vi "CreateReaderFromClass.vi"(0 "ClassPath/LvClassRef":variant, 5 "error in":errorcluster) -> (10 "Is Interface":bool, 14 "ClassReader":refnum<class "ClassReader.lvclass">, 15 "Description":string, 16 "DataFlowClass":bool, 19 "error out":errorcluster)   [LabVIEW 2020, in "ClassReader.lvclass"]
uses:
  <resource>/Framework/Providers/Open_GDS/ClassProviders/Provider_BaseClassInterface/ClassReader_class/ClassReader.lvclass
  <resource>/Framework/Providers/Open_GDS/ClassProviders/Provider_EndevoGOOP300/ClassReaderGOOP300_class/ClassReaderGOOP300.lvclass
  C:/Program Files (x86)/National Instruments/LabVIEW 2020/resource/Framework/Providers/Open_GDS/ClassProviders/Provider_LvNativeClass/ClassReaderNative_class/ClassReaderNative.lvclass
  <resource>/Framework/Providers/Open_GDS/ClassProviders/Provider_EndevoGOOP400/ClassReaderGOOP400_class/ClassReaderGOOP400.lvclass
  <resource>/Framework/Providers/Open_GDS/ClassProviders/Provider_LvNativeClass/ClassReaderNative_class/ClassReaderNative.lvclass
  C:/Program Files (x86)/National Instruments/LabVIEW 2020/resource/Framework/Providers/Open_GDS/ClassProviders/Provider_BaseClassInterface/ClassReader_class/ClassReader.lvclass
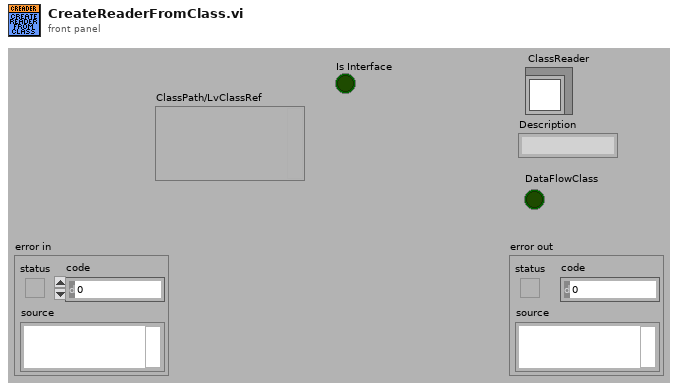
[diagram p1: front panel]
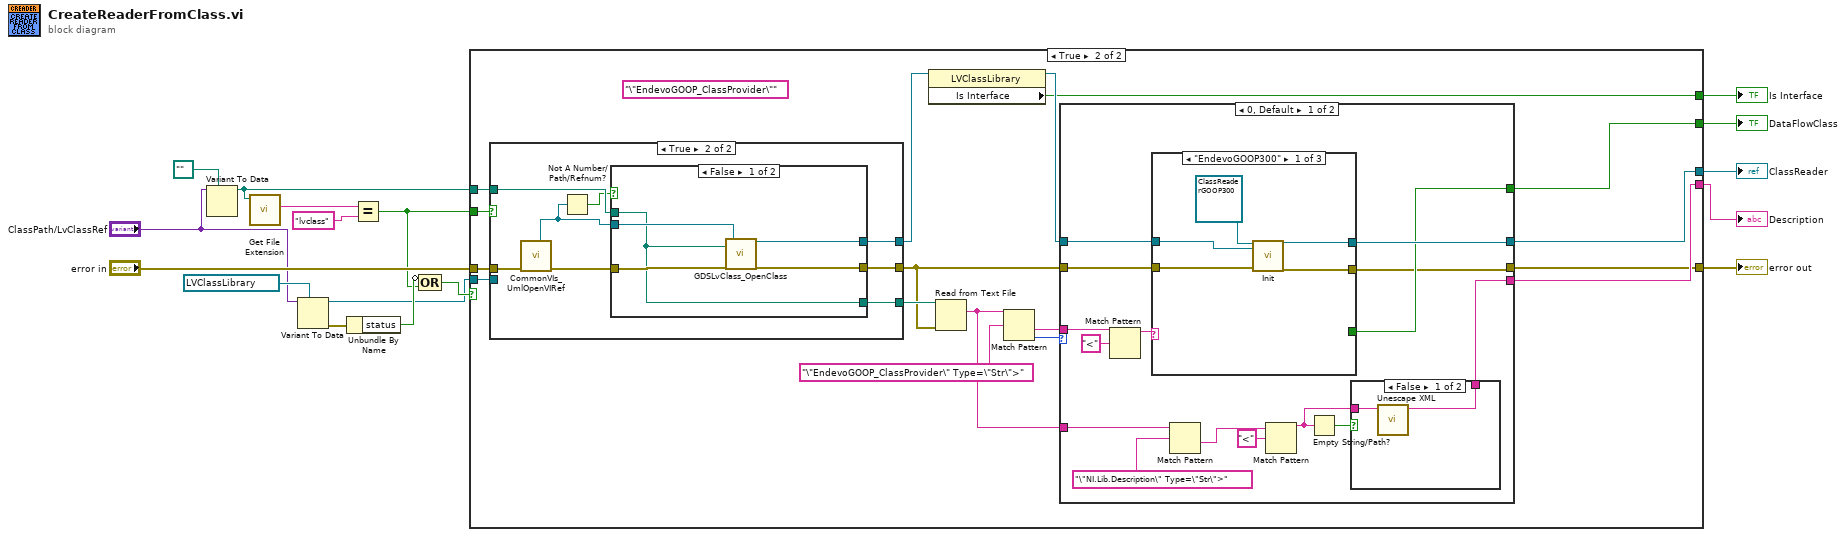
[diagram p0: block diagram]
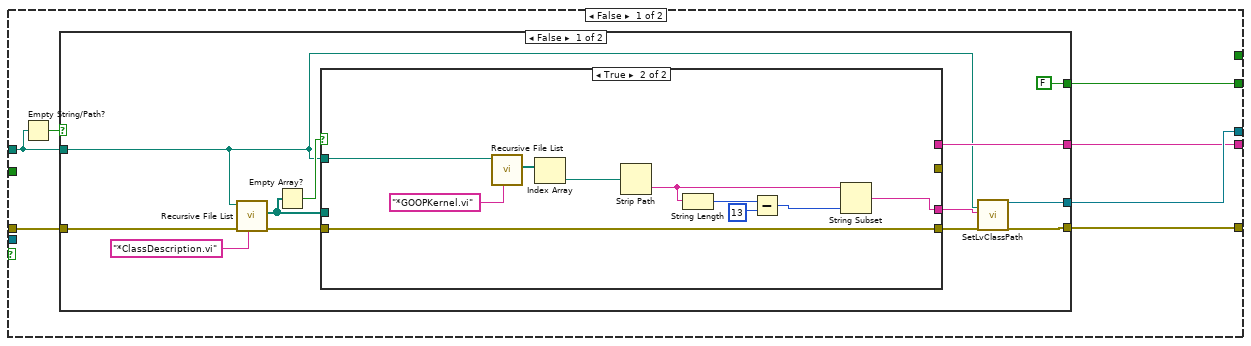
[diagram p2: hidden frame]
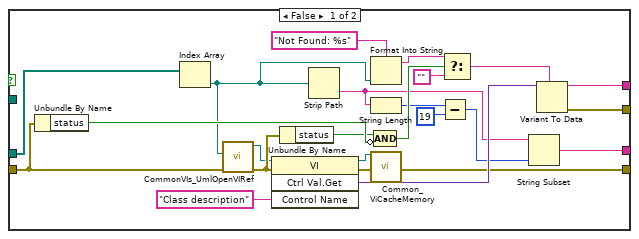
[diagram p3: hidden frame]
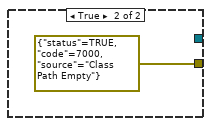
[diagram p4: hidden frame]
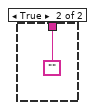
[diagram p5: hidden frame]
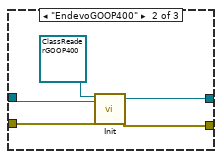
[diagram p6: hidden frame]
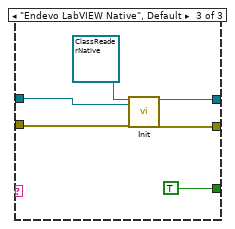
[diagram p7: hidden frame]
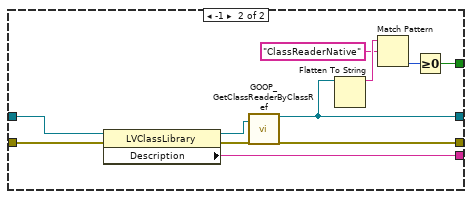
[diagram p8: hidden frame]
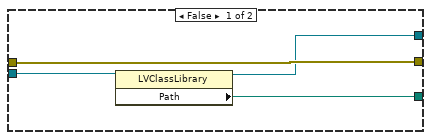
[diagram p9: hidden frame]
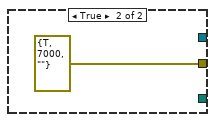
[diagram p10: hidden frame]
diagram:
  n1 = Variant To Data(type=path "", Variant="ClassPath/LvClassRef") -> (data=w5:path)  [unwired: 1 in, 1 out]
  n2 = call <vilib>:"Get File Extension.vi"("file"=w5) -> ("lowercase file extension"=w10:string)  [unwired: 6 in, 4 out]
  n3 = Variant To Data(type=refnum<vi> refnum ("LVClass.Open"), Variant="ClassPath/LvClassRef") -> (data=w4:refnum<vi>, error out=w8:errorcluster)  [unwired: 1 in]
  n4 = Unbundle By Name(w8) -> ("status"=w7:bool)
  n5 = Equal?(x=w10, y="lvclass") -> (x = y?=w3:bool)
  n6 = Compound Arithmetic op=OR(invert w7, w3) -> (w6:bool)
  n7 = case shown="True" w6 {
    tunnel: [w22 w88] -> w17
    tunnel: "error in" -> [w21 w87]
    tunnel: [w24 w82] -> w15
    tunnel: [w23 w86] -> w14
    tunnel: w5 -> [w19 w85]
    tunnel: w4 -> [_ w83]
    tunnel: w3 -> [_ w84]
    tunnel: [w20 w75] -> w2
    tunnel: [_ w72] -> w1
    frame False {
      n8 = Empty String/Path?(string/path=w19) -> (empty?=w18:bool)
      n9 = case shown="False" w18 {
        tunnel: [w36 _] -> w24
        tunnel: [w35 errorcluster {"status"=TRUE, "code"=7000, "source"="Class Path Empty"} ("error out")] -> w23
        tunnel: [w34 _] -> w22
        tunnel: w21 -> [w30 _]
        tunnel: [FALSE _] -> w20
        tunnel: w19 -> [w25 _]
        frame False {
          n10 = call <vilib>:"Recursive File List.vi"("pattern"="*ClassDescription.vi" ("FileSearchPattern"), "error in (no error)"=w30, "Folder Path"=w25) -> ("error out"=w29:errorcluster, "All Files in Dir"=w27:path[])  [unwired: 4 in, 3 out]
          n11 = Empty Array?(array=w27) -> (empty?=w32:bool)
          n12 = case shown="True" w32 {
            tunnel: w29 -> [w46 w70]
            tunnel: [w51 _] -> w34
            tunnel: [w48 w70] -> w33
            tunnel: w27 -> [w47 _]
            tunnel: [w38 w61] -> w31
            tunnel: w25 -> [_ w69]
            tunnel: [w37 _] -> _
            frame False {
              n13 = Unbundle By Name(w46) -> ("status"=w53:bool)
              n14 = Index Array(array=w47) -> (element=w43:path)  [unwired: 1 in]
              n15 = call <resource>:"CommonVIs_UmlOpenVIRef.vi"("error in"=w46, "ViPath/ViName"=w43) -> ("error out"=w45:errorcluster, "vi reference"=w44:refnum<vi>)  [unwired: 6 in, 2 out]
              n16 = invoke class="VI" method="Ctrl Val.Get"(reference=w44, error in=w45, "Control Name"="Class description") -> (reference out=w60:refnum<vi>, error out=w49:errorcluster, "Get Control Value Variant"=w59:variant)  [unwired: 1 in, 1 out]
              n17 = Unbundle By Name(w45) -> ("status"=w52:bool)
              n18 = Strip Path(path=w43) -> (name=w42:string)  [unwired: 1 out]
              n19 = Format Into String(format string="Not Found: %s", w43) -> (resulting string=w57:string)  [unwired: 2 in, 1 out]
              n20 = String Length(string=w42) -> (length=w41:i32)
              n21 = call <resource>:"Common_ ViCacheMemory.vi"("ViRef"=w60, "error in (no error)"=w49) -> ("error out"=w48:errorcluster)  [unwired: 17 in]
              n22 = Compound Arithmetic op=AND(w52, invert w53) -> (w54:bool)
              n23 = Subtract(x=w41, y=19) -> (x-y=w40:i32)
              n24 = Select(t=w57, s=w54, f="") -> (s? t:f=w50:string)
              n25 = String Subset(string=w42, length (rest)=w40) -> (substring=w38:string)  [unwired: 1 in]
              n26 = Variant To Data(type=w50, Variant=w59) -> (data=w51:string, error out=w37:errorcluster)  [unwired: 1 in]
            }
            frame True {
              n27 = call <vilib>:"Recursive File List.vi"("pattern"="*GOOPKernel.vi", "Folder Path"=w69) -> ("All Files in Dir"=w63:path[])  [unwired: 5 in, 4 out]
              n28 = Index Array(array=w63) -> (element=w62:path)  [unwired: 1 in]
              n29 = Strip Path(path=w62) -> (name=w67:string)  [unwired: 1 out]
              n30 = String Length(string=w67) -> (length=w66:i32)
              n31 = Subtract(x=w66, y=13) -> (x-y=w65:i32)
              n32 = String Subset(string=w67, length (rest)=w65) -> (substring=w61:string)  [unwired: 1 in]
            }
          }
          n33 = call <resource>:"SetLvClassPath.vi"("ClassPath"=w25, "ClassName"=w31, "error in (no error)"=w33) -> ("reference out"=w36:refnum<class "ClassReader.lvclass">, "error out"=w35:errorcluster)  [unwired: 15 in]
        }
        frame True {
        }
      }
    }
    frame True {
      (unwired) "\"EndevoGOOP_ClassProvider\"" ("y")
      n34 = case shown="True" w84 {
        tunnel: [w135 w139] -> w74
        tunnel: w87 -> [w137 w145]
        tunnel: [w137 w142] -> w80
        tunnel: w85 -> [_ w143]
        tunnel: w83 -> [w136 _]
        tunnel: [w134 w138] -> w81
        frame False {
          n35 = property class="LVClassLibrary"(reference=w136) -> (reference out=w135:refnum<vi>, "Path"=w134:path)  [unwired: 1 in, 1 out]
        }
        frame True {
          n36 = call <resource>:"CommonVIs_UmlOpenVIRef.vi"("error in"=w145) -> ("error out"=w144:errorcluster, "AppRefOut"=w140:refnum<vi>)  [unwired: 7 in, 2 out]
          n37 = Not A Number/Path/Refnum?(number/path/refnum=w140) -> (NaN/Path/Refnum?=w141:bool)
          n38 = case shown="False" w141 {
            tunnel: [w150 _] -> w139
            tunnel: w144 -> [w149 _]
            tunnel: w143 -> [w146 _]
            tunnel: [w148 errorcluster {"status"=TRUE, "code"=7000, "source"=""} ("error out")] -> w142
            tunnel: w140 -> [w147 _]
            tunnel: [w146 _] -> w138
            frame False {
              n39 = call <resource>:"GDSLvClass_OpenClass.vi"("ClassToOpen"=w146, "error in (no error)"=w149, "Project/ApplicationRef(If empty, currect active project will be used)"=w147) -> ("LVClass.Open"=w150:refnum<vi>, "error out"=w148:errorcluster)  [unwired: 15 in]
            }
            frame True {
            }
          }
        }
      }
      n40 = property class="LVClassLibrary"(reference=w74) -> (reference out=w73:refnum<vi>, "Is Interface"=w72:bool)  [unwired: 1 in, 1 out]
      n41 = Read from Text File(file (use dialog)=w81, error in=w80) -> (text=w76:string)  [unwired: 2 in, 3 out]
      n42 = Match Pattern(string=w76, regular expression="\"EndevoGOOP_ClassProvider\" Type=\"Str\">" ("y")) -> (after substring=w77:string, offset past match=w78:i32)  [unwired: 1 in, 2 out]
      n43 = case shown="0, Default" w78 {
        tunnel: [w94 w133] -> w88
        tunnel: w73 -> [w91 w132]
        tunnel: [w89 w131] -> w86
        tunnel: [w100 w124] -> w82
        tunnel: w80 -> [w90 w128]
        tunnel: w77 -> [w103 _]
        tunnel: w76 -> [w99 _]
        tunnel: [w92 w123] -> w75
        frame 0, Default {
          n44 = Match Pattern(string=w103, regular expression="<") -> (before substring=w101:string)  [unwired: 1 in, 3 out]
          n45 = case shown="\"EndevoGOOP300\"" w101 {
            tunnel: [w111 w113 w121] -> w100
            tunnel: [_ _ TRUE] -> w92
            tunnel: w91 -> [w108 w115 w120]
            tunnel: w90 -> [w110 w116 w118]
            tunnel: [w109 w114 w119] -> w89
            frame "EndevoGOOP300" {
              n46 = call-dynamic "Init.vi"("ClassReaderGOOP300 in"=refnum<class "ClassReaderGOOP300.lvclass"> refnum, "LvClassRef"=w108, "error in (no error)"=w110) -> ("ClassReaderGOOP300 out"=w111:refnum<class "ClassReaderGOOP300.lvclass">, "error out"=w109:errorcluster)  [unwired: 15 in]
            }
            frame "EndevoGOOP400" {
              n47 = call-dynamic "Init.vi"("ClassReaderGOOP300 in"=refnum<class "ClassReaderGOOP400.lvclass"> refnum, "LvClassRef"=w115, "error in (no error)"=w116) -> ("ClassReaderGOOP300 out"=w113:refnum<class "ClassReaderGOOP400.lvclass">, "error out"=w114:errorcluster)  [unwired: 15 in]
            }
            frame "Endevo LabVIEW Native", Default {
              n48 = call-dynamic "Init.vi"("ClassReaderNative in"=refnum<class "ClassReaderNative.lvclass"> refnum, "LvClassRef"=w120, "error in (no error)"=w118) -> ("ClassReaderNative out"=w121:refnum<class "ClassReaderNative.lvclass">, "error out"=w119:errorcluster)  [unwired: 15 in]
            }
          }
          n49 = Match Pattern(string=w99, regular expression="\"NI.Lib.Description\" Type=\"Str\">" ("y")) -> (after substring=w96:string)  [unwired: 1 in, 3 out]
          n50 = Match Pattern(string=w96, regular expression="<") -> (before substring=w93:string)  [unwired: 1 in, 3 out]
          n51 = Empty String/Path?(string/path=w93) -> (empty?=w95:bool)
          n52 = case shown="False" w95 {
            tunnel: [w104 ""] -> w94
            tunnel: w93 -> [w105 _]
            frame False {
              n53 = call <vilib>:"Unescape XML.vi"("XML String In"=w105) -> ("XML String Out"=w104:string)  [unwired: 9 in, 1 out]
            }
            frame True {
            }
          }
        }
        frame -1 {
          n54 = property class="LVClassLibrary"(reference=w132, error in=w128) -> (reference out=w130:refnum<vi>, error out=w129:errorcluster, "Description"=w133:string)
          n55 = call <resource>:"GOOP_GetClassReaderByClassRef.vi"("LVClassLibrary Refnum"=w130, "error in (no error)"=w129) -> ("ClassReaderNative out"=w124:refnum<class "ClassReaderNative.lvclass">, "error out"=w131:errorcluster)  [unwired: 16 in]
          n56 = Flatten To String(anything=w124) -> (data string=w127:string)  [unwired: 3 in, 2 out]
          n57 = Match Pattern(string=w127, regular expression="ClassReaderNative") -> (offset past match=w125:i32)  [unwired: 1 in, 3 out]
          n58 = Greater Or Equal To 0?(x=w125) -> (x >= 0?=w123:bool)
        }
      }
    }
  }
  "Description" <- w17
  "ClassReader" <- w15
  "error out" <- w14
  "DataFlowClass" <- w2
  "Is Interface" <- w1
